vi "Encode enum.vi"(7 "Field Number":i32, 10 "Enumeration":T1, 11 "Buffer in":u8[](array[numeric]) format="%.0x") -> (3 "Buffer":u8[](array[numeric]) format="%.0x")   [LabVIEW 2020, in "ServiceType.lvlib"]
uses:
  ServiceType.lvlib
  lv-protoc/LV-Proto/LV-Proto.lvlib
  lv-protoc/LV-Proto/Wire Type.ctl
  Enumeration.ctl
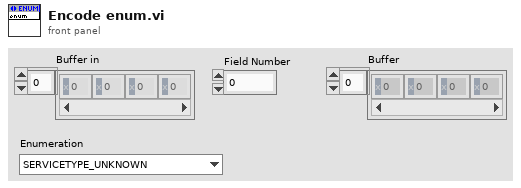
[diagram p1: front panel]
types:
  T1 = typedef "ServiceType.lvlib/Enumeration.ctl" = enum16{"SERVICETYPE_UNKNOWN", "SERVICETYPE_TCPSERVER", "SERVICETYPE_HTTPSERVER"}
  T2 = typedef "LV-Proto.lvlib/Wire Type.ctl" = enum8{"VARINT", "I64", "LEN", "SGROUP (Deprecated)", "EGROUP (Deprecated)", "I32"}
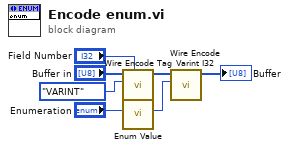
[diagram p0: block diagram]
diagram:
  n1 = call "Wire Encode Tag.vi"("Field Number"="Field Number", "Wire Type"=Wire_Type."VARINT", "Buffer in"="Buffer in") -> ("Buffer"=w3:u8[])  [unwired: 8 in]
  n2 = call "Enum Value.vi"("Enumeration"="Enumeration") -> ("Value"=w2:i32)  [unwired: 10 in]
  n3 = call "Wire Encode Varint I32.vi"("I32"=w2, "Buffer in"=w3) -> ("Buffer"=→"Buffer":u8[])  [unwired: 9 in]
